vi "StartMaster.vi"(8 "error in (no error)":errorcluster, 11 "Tasks In":refnum<k21>[](array[refnum])) -> (0 "error out":errorcluster, 3 "Tasks Out":refnum<k21>[](array[refnum]))   [LabVIEW 2011]
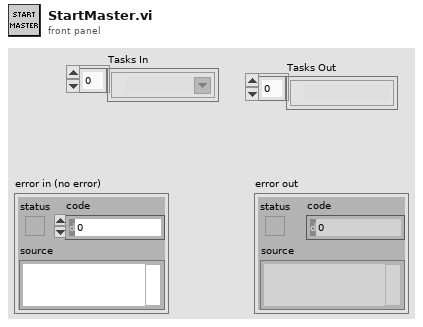
[diagram p1: front panel]
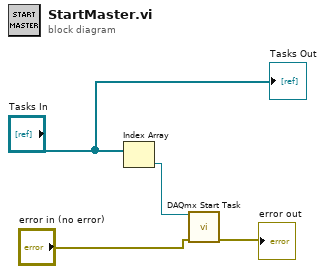
[diagram p0: block diagram]
diagram:
  n1 = Index Array(array="Tasks In") -> (element=w4:refnum<k21>)  [unwired: 1 in]
  n2 = call <vilib>:"DAQmx Start Task.vi"("task/channels in"=w4, "error in"="error in (no error)") -> ("error out"=→"error out":errorcluster)  [unwired: 12 in, 1 out]
  "Tasks Out" <- "Tasks In"
